vi "Handle Open Word or Excel File.vi"(6 "previous error":errorcluster, 8 "file error":errorcluster) -> (0 "error out":errorcluster, 3 "Error 5 or 6?":bool)   [LabVIEW 2010]
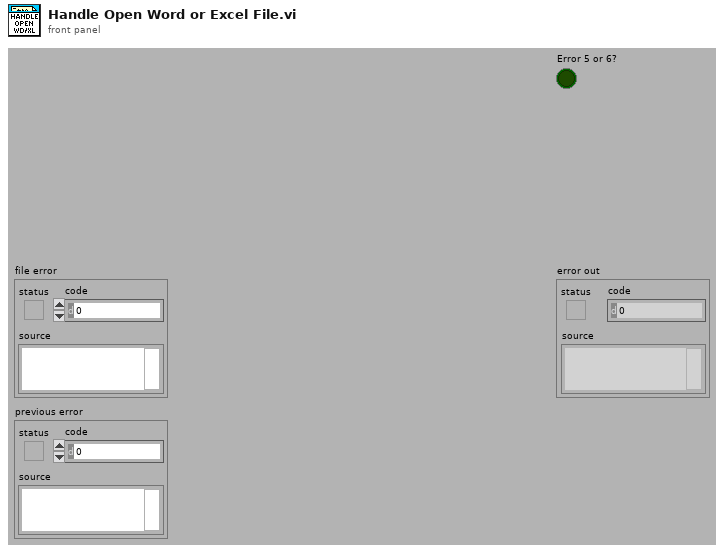
[diagram p1: front panel]
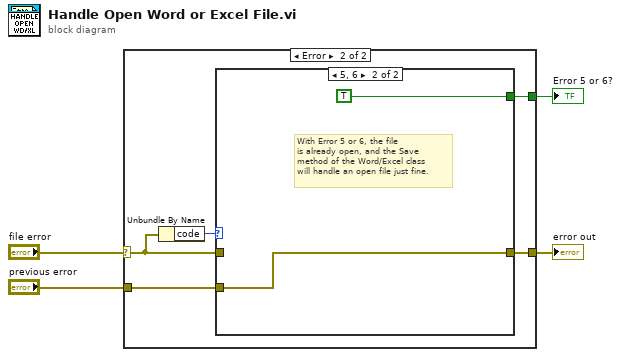
[diagram p0: block diagram]
diagram:
  n1 = case shown="Error" "file error" {
    selector: "file error" -> [w5 w9]
    tunnel: [w5 w8] -> w3
    tunnel: "previous error" -> [_ w7]
    tunnel: [_ w6] -> w1
    frame No Error {
      # "If No Error, the file is not open.  Proceed as normal."
    }
    frame Error {
      n2 = Unbundle By Name(w9) -> ("code"=w10:i32)
      n3 = case shown="5, 6" w10 {
        tunnel: w9 -> [w11 _]
        tunnel: [w11 w12] -> w8
        tunnel: w7 -> [_ w12]
        tunnel: [_ TRUE] -> w6
        frame Default {
          # "Don't do anything special for errors other\nthan Error 5 or 6.  Just pass them through."
        }
        frame 5, 6 {
          # "With Error 5 or 6, the file\nis already open, and the Save\nmethod of the Word/Excel class\nwill handle an open file just fine."
        }
      }
    }
  }
  "error out" <- w3
  "Error 5 or 6?" <- w1
